vi "Teleop.vi"(0 "Call Context":T2, 1 "Match Info":T1={"Autonomous Elapsed Seconds"=0.0, "TeleOp Elapsed Seconds"=0.0, "Disabled Elapsed Seconds"=0.0, "Visited Autonomous"=FALSE, "Visited TeleOp"=FALSE, "Visited Disabled"=FALSE, "Autonomous Settings"={"Autonomous Style"=enum."Independent", "VI Refnum"=refnum}}) -> ()   [LabVIEW 2017]
doc: "This VI is called for each TeleOp packet received from the DS where the robot is not disabled. It is often used to read from the joysticks and update I/O or to update setpoints for timed control loops. It should complete and return within 20 milliseconds or it may miss DS packets."
uses:
  <vilib>/Rock Robotics/WPI/DriverStation/WPI_DriverStationDerivedRobotMode.ctl
  <vilib>/Rock Robotics/WPI/DriverStation/WPI_DriverStationMatch Info.ctl
  <vilib>/Rock Robotics/WPI/Utilities/WPI_GetSetVariantRefNum.vi
  <vilib>/Rock Robotics/Network Tables/NT Write Boolean Array.vi
  <vilib>/Rock Robotics/Network Tables/NT Write Numeric Array.vi
  <vilib>/Rock Robotics/Network Tables/NT Read Boolean.vi
  <vilib>/Rock Robotics/Network Tables/NT Read Number.vi
panel:
  out "Compressor Running":bool
  out "Enabled":bool
  out "Sample Slider 0":dbl(slide) scale=0.0..5.0
  out "Sample Boolean 1":bool
  out "Sample Boolean 0":bool
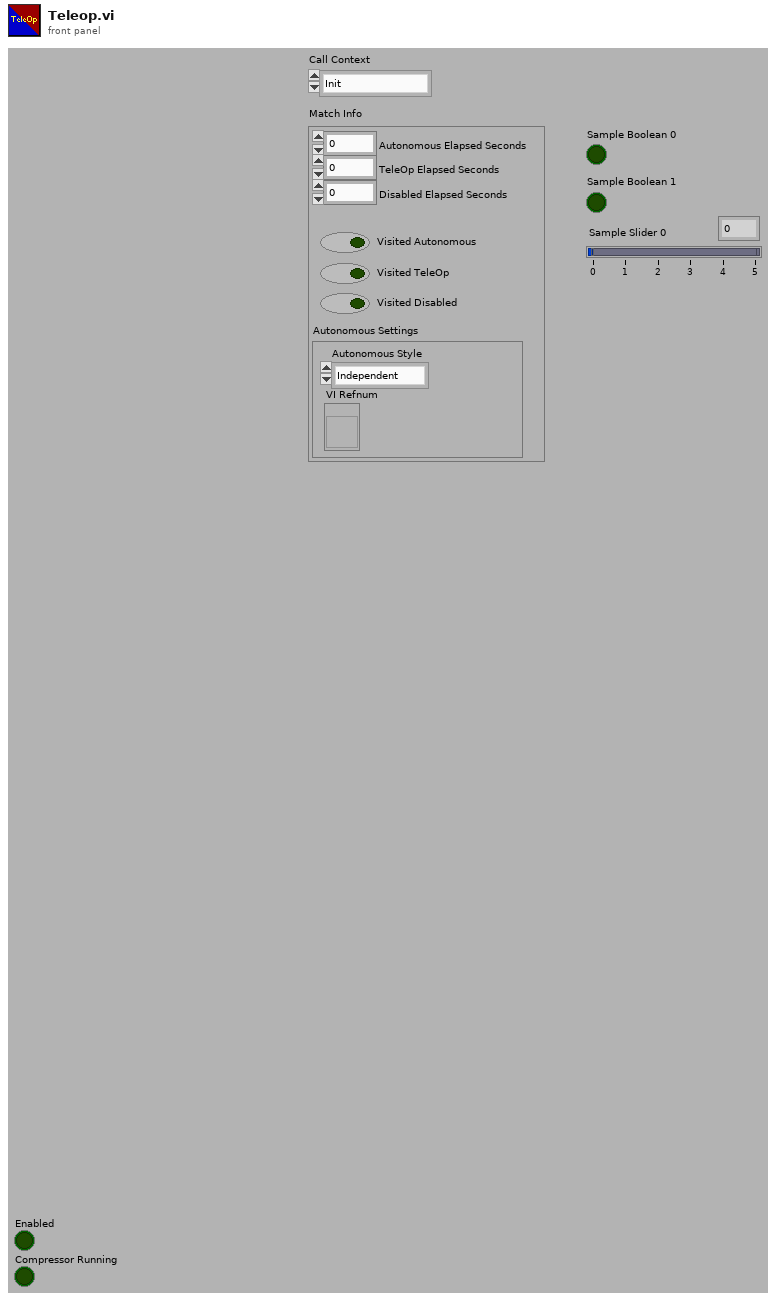
[diagram p1: front panel]
types:
  T1 = typedef "WPI_DriverStationMatch Info.ctl" = cluster{"Autonomous Elapsed Seconds":dbl, "TeleOp Elapsed Seconds":dbl, "Disabled Elapsed Seconds":dbl, "Visited Autonomous":bool, "Visited TeleOp":bool, "Visited Disabled":bool, "Autonomous Settings":cluster{"Autonomous Style":enum16{"Iterative", "Independent"}, "VI Refnum":refnum<vi>}}
  T2 = typedef "WPI_DriverStationDerivedRobotMode.ctl" = enum16{"Init", "Execute", "Stop"}
  T3 = typedef "WPI_CompressorDevRef.ctl" = cluster{"DevStatus":errorcluster, "Pneumatics Control Module":u8}
  T4 = typedef "WPI_JoystickDevRef.ctl" = cluster{"Device":T5}
  T5 = typedef "WPI_JoystickDeviceEnum.ctl" = enum16{"USB 0", "USB 1", "USB 2", "USB 3", "USB 4", "USB 5"}
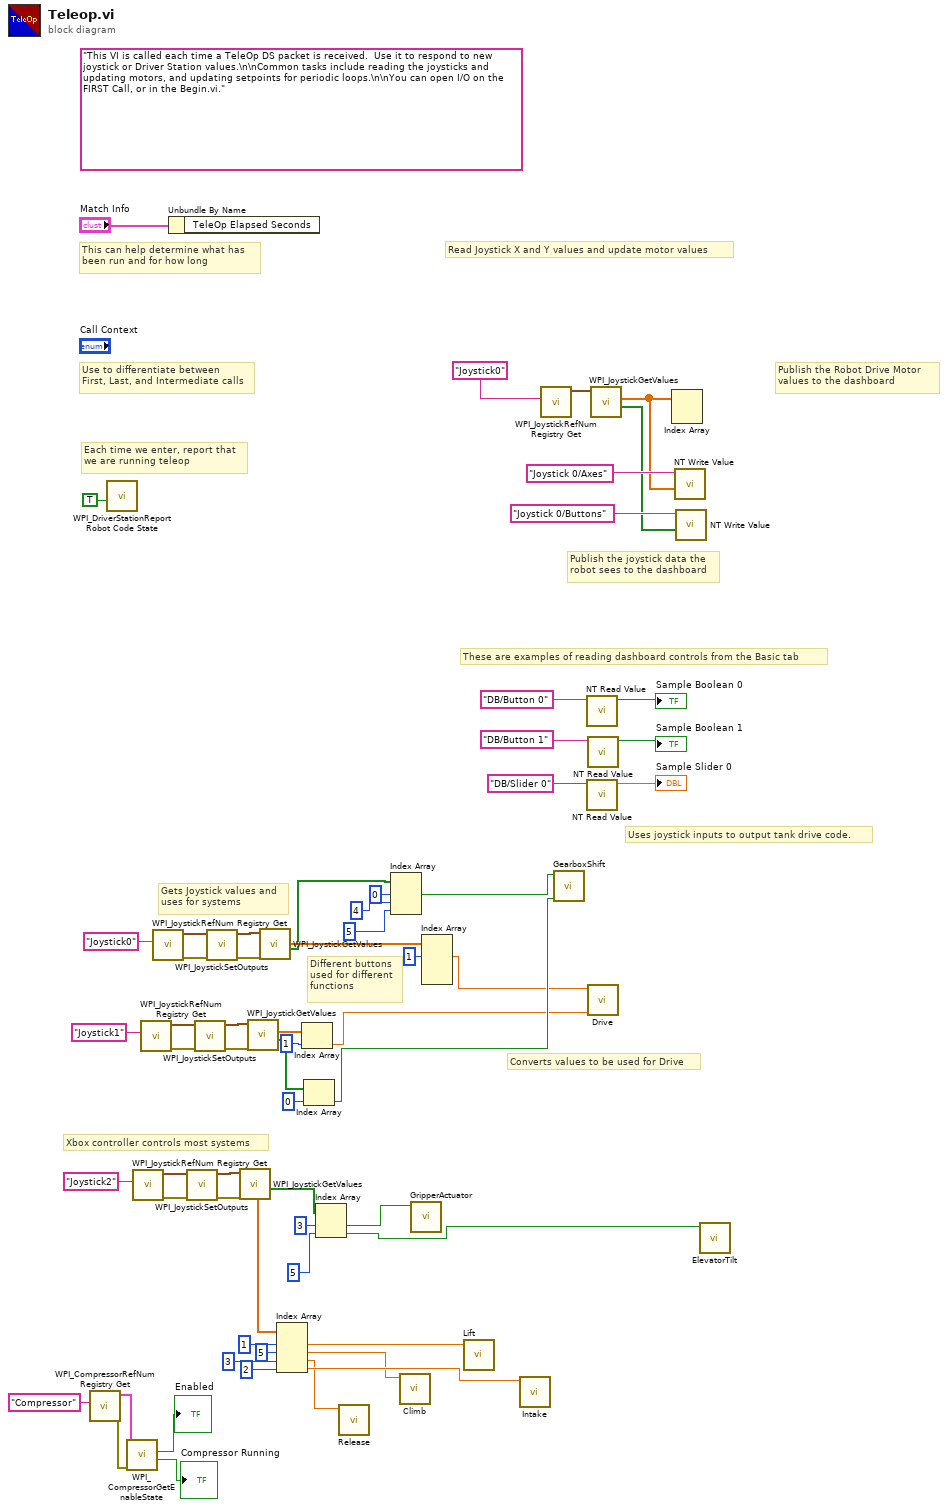
[diagram p0: block diagram]
diagram:
  (unwired) "This VI is called each time a TeleOp DS packet is received.  Use it to respond to new joystick or Driver Station values.\n\nCommon tasks include reading the joysticks and updating motors, and updating setpoints for periodic loops.\n\nYou can open I/O on the FIRST Call, or in the Begin.vi."
  # "Xbox controller controls most systems"
  # "Converts values to be used for Drive"
  # "Different buttons\nused for different\nfunctions"
  # "Gets Joystick values and\nuses for systems"
  # "Uses joystick inputs to output tank drive code."
  # "These are examples of reading dashboard controls from the Basic tab"
  # "Publish the Robot Drive Motor\nvalues to the dashboard"
  # "Publish the joystick data the\nrobot sees to the dashboard"
  # "Each time we enter, report that\nwe are running teleop"
  # "Use to differentiate between\nFirst, Last, and Intermediate calls"
  # "This can help determine what has\nbeen run and for how long"
  # "Read Joystick X and Y values and update motor values"
  n1 = call <vilib>:"WPI_CompressorRefNum Registry Get.vi"("refnum name"="Compressor") -> ("error out"=w23:errorcluster, "CompressorDevRef"=w22:T3)  [unwired: 9 in]
  n2 = call <vilib>:"WPI_DriverStationReport Robot Code State.vi"("TeleOp"=TRUE ("Autonomous")) -> ()  [unwired: 10 in, 1 out]
  n3 = call <vilib>:"WPI_CompressorGetEnableState.vi"("error in (no error)"=w23, "CompressorDevRef"=w22) -> ("Compressor Running"=→"Compressor Running":bool, "Enabled"=→"Enabled":bool)  [unwired: 6 in, 2 out]
  n4 = call <vilib>:"WPI_JoystickRefNum Registry Get.vi"("refnum name"="Joystick2") -> ("error out"=w29:errorcluster, "JoystickDevRef"=w31:T4)  [unwired: 1 in, 8 out]
  n5 = call <vilib>:"WPI_JoystickRefNum Registry Get.vi"("refnum name"="Joystick1") -> ("error out"=w40:errorcluster, "JoystickDevRef"=w38:T4)  [unwired: 1 in, 8 out]
  n6 = call <vilib>:"WPI_JoystickRefNum Registry Get.vi"("refnum name"="Joystick0") -> ("error out"=w43:errorcluster, "JoystickDevRef"=w45:T4)  [unwired: 1 in, 8 out]
  n7 = Unbundle By Name("Match Info") -> ()  [unwired: 1 out]
  n8 = call <vilib>:"WPI_JoystickSetOutputs.vi"("error in (no error)"=w29, "JoystickDevRef"=w31) -> ("error out"=w28:errorcluster, "JoystickDevRef"=w30:T4)  [unwired: 8 in]
  n9 = call <vilib>:"WPI_JoystickSetOutputs.vi"("error in (no error)"=w40, "JoystickDevRef"=w38) -> ("error out"=w41:errorcluster, "JoystickDevRef"=w39:T4)  [unwired: 8 in]
  n10 = call <vilib>:"WPI_JoystickSetOutputs.vi"("error in (no error)"=w43, "JoystickDevRef"=w45) -> ("error out"=w42:errorcluster, "JoystickDevRef"=w44:T4)  [unwired: 8 in]
  n11 = call <vilib>:"WPI_JoystickGetValues.vi"("error in (no error)"=w28, "JoystickDevRef"=w30) -> ("Buttons"=w27:bool[], "Axes"=w24:dbl[])  [unwired: 5 in, 3 out]
  n12 = call <vilib>:"WPI_JoystickGetValues.vi"("error in (no error)"=w41, "JoystickDevRef"=w39) -> ("Buttons"=w17:bool[], "Axes"=w36:dbl[])  [unwired: 5 in, 3 out]
  n13 = call <vilib>:"WPI_JoystickGetValues.vi"("error in (no error)"=w42, "JoystickDevRef"=w44) -> ("Buttons"=w33:bool[], "Axes"=w48:dbl[])  [unwired: 5 in, 3 out]
  n14 = Index Array(array=w24, index #1=1 ("index"), index #2=5 ("index"), index #3=3 ("index"), index #4=2 ("index")) -> (element #1=w5:dbl, element #2=w3:dbl, element #3=w4:dbl, element #4=w6:dbl)
  n15 = Index Array(array=w36, index=1) -> (element=w13:dbl)
  n16 = Index Array(array=w17, index=0) -> (element=w15:bool)
  n17 = Index Array(array=w27, index #1=3 ("index"), index #2=5 ("index")) -> (element #1=w8:bool, element #2=w2:bool)
  n18 = call "Release.vi"("Release"=w4) -> ()  [unwired: 11 in]
  n19 = Index Array(array=w33, index #1=0 ("index"), index #2=4 ("index"), index #3=5 ("index")) -> (element #1=w18:bool)  [unwired: 2 out]
  n20 = call "Climb.vi"("EFfort"=w3) -> ()  [unwired: 11 in]
  n21 = call "GripperActuator.vi"("Up"=w8) -> ()  [unwired: 11 in]
  n22 = Index Array(array=w48, index #1=1 ("index")) -> (element #1=w14:dbl)  [unwired: 3 in, 3 out]
  n23 = call "Lift.vi"("Effort"=w5) -> ()  [unwired: 11 in]
  n24 = call "Intake.vi"("Intake"=w6) -> ()  [unwired: 11 in]
  n25 = call <vilib>:"WPI_JoystickRefNum Registry Get.vi"("refnum name"="Joystick0") -> ("JoystickDevRef"=w60:T4)  [unwired: 1 in, 9 out]
  n26 = call "GearboxShift.vi"("Gear2"=w15, "Gear1"=w18) -> ()  [unwired: 10 in]
  n27 = call-poly <vilib>:"NT Read Value.vi"("Name"="DB/Button 0" ("refnum name")) -> ("Boolean"=→"Sample Boolean 0":bool)  [unwired: 9 in, 1 out]
  n28 = call-poly <vilib>:"NT Read Value.vi"("Name"="DB/Slider 0" ("refnum name")) -> ("Numeric"=→"Sample Slider 0":dbl)  [unwired: 9 in, 1 out]
  n29 = call-poly <vilib>:"NT Read Value.vi"("Name"="DB/Button 1" ("refnum name")) -> ("Boolean"=→"Sample Boolean 1":bool)  [unwired: 9 in, 1 out]
  n30 = call "Drive.vi"("Drive R"=w13, "Drive L"=w14) -> ()  [unwired: 10 in]
  n31 = call <vilib>:"WPI_JoystickGetValues.vi"("JoystickDevRef"=w60) -> ("Buttons"=w55:bool[], "Axes"=w56:dbl[])  [unwired: 6 in, 3 out]
  n32 = Index Array(array=w56) -> ()  [unwired: 2 in, 2 out]
  n33 = call-poly <vilib>:"NT Write Value.vi"("Numeric Array"=w56, "Name"="Joystick 0/Axes") -> ()  [unwired: 9 in, 1 out]
  n34 = call-poly <vilib>:"NT Write Value.vi"("Boolean Array"=w55, "Name"="Joystick 0/Buttons") -> ()  [unwired: 9 in, 1 out]
  n35 = call "ElevatorTilt.vi"("Up"=w2) -> ()  [unwired: 11 in]
